vi "Begin.vi"(8 "error in":errorcluster) -> (0 "error out":errorcluster)   [LabVIEW 2014]
doc: "Called before other user functions, this VI is expected to open initial I/O refnums, load in file data, and do all program initialization. Notice that the <B>error out</B> terminal is simply used for data flow. Wiring it to other structures or subVIs ensures that this VI runs first."
uses:
  <vilib>/Rock Robotics/WPI/SafetyOutput/WPI_SafetyOutputConfigMenu.ctl
  <vilib>/Rock Robotics/WPI/DriverStation/WPI_DriverStationRobotMode2.ctl
  <vilib>/Rock Robotics/WPI/Joystick/WPI_JoystickDeviceEnum.ctl
  <vilib>/Rock Robotics/SystemInterfaces/DIO/FPGA_DIOPWMChannel.ctl
  <vilib>/Rock Robotics/SystemInterfaces/AI/FPGA_AIChannel.ctl
  <vilib>/Rock Robotics/SystemInterfaces/Typedef/FPGA_TypedefAnalogModule.ctl
  <vilib>/Rock Robotics/WPI/SerialPort/WPI_SerialPort.ctl
  <vilib>/Rock Robotics/SystemInterfaces/DIO/FPGA_DIOChannel.ctl
  <vilib>/Rock Robotics/WPI/Encoder/WPI_EncoderType.ctl
  Robot Global Data.vi
  <vilib>/Rock Robotics/Network Tables/SD Write String Array.vi
  <vilib>/Rock Robotics/WPI/MotorControl/WPI_MotorControlOpen Talon.vi
  <vilib>/Rock Robotics/WPI/Counter/WPI_CounterDigitalInputToDigitalSource.vi
  <vilib>/Rock Robotics/WPI/RobotDrive/WPI_RobotDriveOpen4MotorWithTalon.vi
  <vilib>/Rock Robotics/SystemInterfaces/spilib/spi_bus.ctl
  <vilib>/Rock Robotics/WPI/SPI/WPI_SPIMode.ctl
  <vilib>/Rock Robotics/SystemInterfaces/Typedef/FPGA_TypedefDigitalModule.ctl
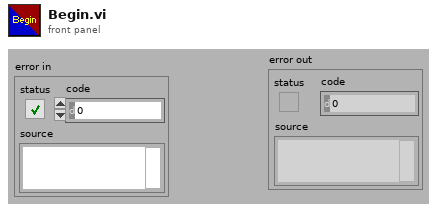
[diagram p1: front panel]
types:
  T1 = typedef "WPI_JoystickDeviceEnum.ctl" = enum16{"USB 0", "USB 1", "USB 2", "USB 3", "USB 4", "USB 5"}
  T2 = typedef "WPI_EncoderType.ctl" = enum16{"1x", "2x", "4x"}
  T3 = typedef "FPGA_DIOChannel.ctl" = enum8{"DIO 0", "DIO 1", "DIO 2", "DIO 3", "DIO 4", "DIO 5", "DIO 6", "DIO 7", "DIO 8", "DIO 9", "DIO MXP 0", "DIO MXP 1", "DIO MXP 2", "DIO MXP 3", "DIO MXP 4", "DIO MXP 5", "DIO MXP 6", "DIO MXP 7", "DIO MXP 8", "DIO MXP 9", "DIO MXP 10", "DIO MXP 11", "DIO MXP 12", "DIO MXP 13", "DIO MXP 14", "DIO MXP 15", "Invalid"}
  T4 = typedef "FPGA_DIOPWMChannel.ctl" = enum8{"PWM 0", "PWM 1", "PWM 2", "PWM 3", "PWM 4", "PWM 5", "PWM 6", "PWM 7", "PWM 8", "PWM 9", "PWM MXP 0", "PWM MXP 1", "PWM MXP 2", "PWM MXP 3", "PWM MXP 4", "PWM MXP 5", "PWM MXP 6", "PWM MXP 7", "PWM MXP 8", "PWM MXP 9", "Invalid"}
  T5 = typedef "WPI_SerialPort.ctl" = enum16{"Onboard RS-232", "MXP TTL"}
  T6 = typedef "FPGA_AIChannel.ctl" = enum8{"AI 0", "AI 1", "AI 2", "AI 3", "AI MXP 0", "AI MXP 1", "AI MXP 2", "AI MXP 3", "Invalid"}
  T7 = typedef "FPGA_TypedefAnalogModule.ctl" = enum16{"Controller 1"}
  T8 = typedef "WPI_DriverStationRobotMode2.ctl" = enum16{"Autonomous Disabled", "Autonomous Enabled", "Teleop Disabled", "Teleop Enabled", "Disconnected", "Finish", "Test Disabled", "Test Enabled", "Emergency Stopped"}
  T9 = typedef "WPI_SafetyOutputConfigMenu.ctl" = enum16{"Enable", "Disable"}
  T10 = typedef "FPGA_TypedefDigitalModule.ctl" = enum16{"Controller 1"}
  T11 = typedef "WPI_SPIMode.ctl" = enum16{"Mode 0 (Clk Idle Low,Sample on Leading)", "Mode 1 (Clk Idle Low,Sample on Trailing)", "Mode 2 (Clk Idle High,Sample on Leading)", "Mode 3 (Clk Idle High,Sample on Trailing)"}
  T12 = typedef "spi_bus.ctl" = enum16{"SPI On-Board, CS0", "SPI On-Board, CS1", "SPI On-Board, CS2", "SPI On-Board, CS3", "SPI MXP", "Invalid"}
  T13 = typedef "WPI_SPIDevRef.ctl" = cluster{"DevStatus":errorcluster, "Handle":i32, "Controller":T10, "SPI Bus":T12}
  T14 = typedef "WPI_SerialPortRef.ctl" = cluster{"DevStatus":errorcluster, "Serial Port Name":refnum<visa-resource-name>}
  T15 = typedef "WPI_DigitalInputDevRef.ctl" = cluster{"DevStatus":errorcluster, "DIO Channel":T3, "Controller":T10}
  T16 = typedef "WPI_JoystickDevRef.ctl" = cluster{"Device":T1}
  T17 = typedef "WPI_RobotDriveDevRef.ctl" = cluster{"DevStatus":errorcluster, "Motors[]":T18[], "Square Inputs":bool, "Max Output":dbl}
  T18 = typedef "WPI_MotorControlDeviceRef.ctl" = cluster{"DeviceStatus":errorcluster, "Type":T19, "PWM":cluster{"Controller":T10, "PWM Channel":T4, "DeadBand":T20}, "CAN":cluster{"Device Number":u8, "Control Mode":T21, "Semaphore":T22, "Max Vout":dbl, "TalonSRX Control Mode":T23}, "Invert":bool, "TransformRef":T24, "InvTransformRef":T24}
  T19 = typedef "WPI_MotorControlType.ctl" = enum16{"PWM", "CAN", "CANTalonSRX"}
  T20 = typedef "WPI_PWMDeadband.ctl" = cluster{"Name":string, "maxPositivePwm":i32, "minPositivePwm":i32, "centerPwm":i32, "maxNegativePwm":i32, "minNegativePwm":i32, "angularRange":u16}
  T21 = typedef "WPI_CANJaguar_ControlMode.ctl" = enum8{"Percent VBus", "Current", "Speed", "Position", "Voltage"}
  T22 = typedef "Semaphore RefNum" = refnum<k1>
  T23 = typedef "WPI_CANTalonSRX_APIControlMode.ctl" = enum8{"Percent VBus", "Speed", "Position", "Slave", "Unchanged / Invalid"}
  T24 = typedef "WPI_PWMTransform_ConPane.ctl" = refnum<vi>
  T25 = typedef "FPGA_CounterEncoderSourceConvertionLVSourceType.ctl" = cluster{"DevStatus":errorcluster, "AnalogTriggerMode?":bool, "DigitalMode":cluster{"Controller":T10, "DIO Channel":T26}, "AnalogTriggerMode":cluster{"AnalogTriggerIndex":T27, "OutputType":T28}}
  T26 = typedef "FPGA_DIODigitalSourceChannel.ctl" = enum8{"DIO 0", "DIO 1", "DIO 2", "DIO 3", "DIO 4", "DIO 5", "DIO 6", "DIO 7", "DIO 8", "DIO 9", "DIO MXP 0", "DIO MXP 1", "DIO MXP 2", "DIO MXP 3", "DIO MXP 4", "DIO MXP 5", "DIO MXP 6", "DIO MXP 7", "DIO MXP 8", "DIO MXP 9", "DIO MXP 10", "DIO MXP 11", "DIO MXP 12", "DIO MXP 13", "DIO MXP 14", "DIO MXP 15", "Disabled"}
  T27 = typedef "FPGA_AnalogTriggerIndex.ctl" = enum8{"Trig 0", "Trig 1", "Trig 2", "Trig 3", "Trig 4", "Trig 5", "Trig 6", "Trig 7", "Invalid"}
  T28 = typedef "FPGA_AnalogTriggerOutType.ctl" = enum16{"InWindow", "TriggerState", "Rising", "Falling"}
  T29 = typedef "WPI_EncoderDevRef.ctl" = cluster{"DevStatus":errorcluster, "EncoderIndex":T30, "CounterIndex":T31, "DistancePerCount":dbl, "Decoding Type":T2}
  T30 = typedef "FPGA_EncoderIdx.ctl" = enum8{"Enc 0", "Enc 1", "Enc 2", "Enc 3", "Enc 4", "Enc 5", "Enc 6", "Enc 7", "Invalid"}
  T31 = typedef "FPGA_CounterCtrSystemIndex.ctl" = enum8{"Ctr 0", "Ctr 1", "Ctr 2", "Ctr 3", "Ctr 4", "Ctr 5", "Ctr 6", "Ctr 7", "Invalid"}
  T32 = typedef "WPI_PotentiometerDevRef.ctl" = cluster{"DevStatus":errorcluster, "Controller":T7, "Analog Channel":T6, "Invert Output":bool}
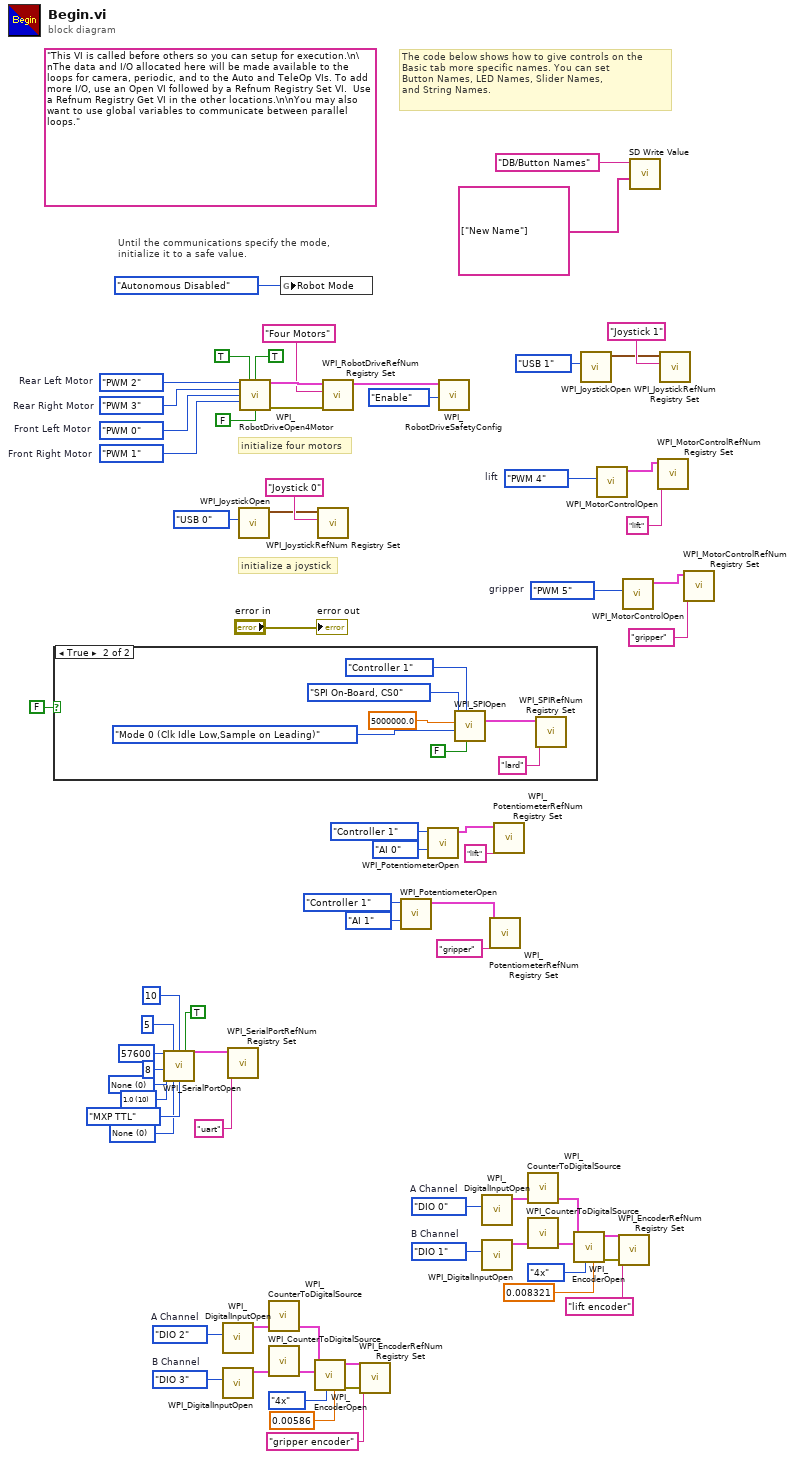
[diagram p0: block diagram]
diagram:
  w19 = FPGA_DIOChannel."DIO 3"  # B Channel
  w18 = FPGA_DIOChannel."DIO 2"  # A Channel
  w29 = FPGA_DIOChannel."DIO 1"  # B Channel
  w28 = FPGA_DIOChannel."DIO 0"  # A Channel
  w32 = FPGA_DIOPWMChannel."PWM 5"  # gripper
  w35 = FPGA_DIOPWMChannel."PWM 4"  # lift
  w38 = u16 0 items=["None", "XON/XOFF", "RTS/CTS", "XON/XOFF & RTS/CTS", "DTR/DSR", "XON/XOFF & DTR/DSR"] ("Flow Control")
  w42 = u16 10 items=["1.0"=10, "1.5"=15, "2.0"=20] ("Stop Bits")
  w43 = u16 0 items=["None", "Odd", "Even", "Mark", "Space"] ("Parity")
  w58 = FPGA_DIOPWMChannel."PWM 1"  # Front Right Motor
  w59 = FPGA_DIOPWMChannel."PWM 0"  # Front Left Motor
  w60 = FPGA_DIOPWMChannel."PWM 3"  # Rear Right Motor
  w61 = FPGA_DIOPWMChannel."PWM 2"  # Rear Left Motor
  (unwired) "This VI is called before others so you can setup for execution.\n\nThe data and I/O allocated here will be made available to the loops for camera, periodic, and to the Auto and TeleOp VIs. To add more I/O, use an Open VI followed by a Refnum Registry Set VI.  Use a Refnum Registry Get VI in the other locations.\n\nYou may also want to use global variables to communicate between parallel loops."
  # "The code below shows how to give controls on the\nBasic tab more specific names. You can set\nButton Names, LED Names, Slider Names,\nand String Names."
  # "initialize a joystick"
  # "Until the communications specify the mode,\ninitialize it to a safe value."
  # "initialize four motors"
  n1 = case shown="True" FALSE {
    frame False {
    }
    frame True {
      n2 = call <vilib>:"WPI_SPIOpen.vi"("Chip Select Active High (F)"=FALSE, "Controller"=FPGA_TypedefDigitalModule."Controller 1", "Mode (3)"=WPI_SPIMode."Mode 0 (Clk Idle Low,Sample on Leading)", "Clock Rate (Hz)"=5000000.0, "SPI Bus"=spi_bus."SPI On-Board, CS0") -> ("SPIDevRef"=w72:T13)  [unwired: 5 in, 1 out]
      n3 = call <vilib>:"WPI_SPIRefNum Registry Set.vi"("refnum name"="lard", "SPIDevRef"=w72) -> ()  [unwired: 8 in, 2 out]
    }
  }
  n4 = call <vilib>:"WPI_SerialPortOpen.vi"("Baud Rate"=u32 57600, "Timeout Value (ms)"=u32 5, "Termination Char (0xA = '\\n' = LF)"=u8 10 ("Termination Char (0xA = '\\n' = LF)"), "Enable Termination Char? (T)"=TRUE, "Data Bits"=u16 8, "Parity"=w43, "Stop Bits"=w42, "Flow Control"=w38, "Serial Port"=WPI_SerialPort."MXP TTL") -> ("SerialPortRef"=w41:T14)  [unwired: 5 in, 1 out]
  n5 = call <vilib>:"WPI_DigitalInputOpen.vi"("DIO Channel"=w18) -> ("DigitalInputDevRef"=w15:T15)  [unwired: 2 in, 8 out]
  n6 = call <vilib>:"WPI_DigitalInputOpen.vi"("DIO Channel"=w19) -> ("DigitalInputDevRef"=w16:T15)  [unwired: 2 in, 8 out]
  n7 = call <vilib>:"WPI_SerialPortRefNum Registry Set.vi"("refnum name"="uart", "SerialPortRef"=w41) -> ()  [unwired: 8 in, 2 out]
  n8 = call <vilib>:"WPI_JoystickOpen.vi"("JoystickDevice"=WPI_JoystickDeviceEnum."USB 0") -> ("JoystickDevRef"=w63:T16)  [unwired: 10 in]
  n9 = call-poly <vilib>:"WPI_RobotDriveOpen4Motor.vi"("Rear Left Motor"=w61, "Rear Left Motor Inverted"=TRUE, "Rear Right Motor Inverted"=TRUE, "Rear Right Motor"=w60, "Front Left Motor"=w59, "Front Right Motor"=w58, "Front Right Motor Inverted"=FALSE) -> ("RobotDriveDevRef"=w70:T17, "error out"=w68:errorcluster)  [unwired: 7 in]
  n10 = call-poly <vilib>:"WPI_CounterToDigitalSource.vi"("DigitalInputDevRef"=w15) -> ("Digital Source"=w14:T25)  [unwired: 6 out]
  n11 = call-poly <vilib>:"WPI_CounterToDigitalSource.vi"("DigitalInputDevRef"=w16) -> ("Digital Source"=w17:T25)  [unwired: 6 out]
  n12 = global write "Robot Global Data.vi" "Robot Mode"(WPI_DriverStationRobotMode2."Autonomous Disabled" ("Robot Mode")) -> ()
  n13 = call <vilib>:"WPI_EncoderOpen.vi"("DistancePerCount"=0.00586, "Decoding Type"=WPI_EncoderType."4x", "BSource"=w17, "ASource"=w14) -> ("error out"=w13:errorcluster, "EncoderDevRef"=w12:T29)  [unwired: 4 in, 2 out]
  n14 = call <vilib>:"WPI_JoystickRefNum Registry Set.vi"("refnum name"="Joystick 0", "JoystickDevRef"=w63) -> ()  [unwired: 8 in, 2 out]
  n15 = call <vilib>:"WPI_RobotDriveRefNum Registry Set.vi"("error in (no error)"=w68, "refnum name"="Four Motors", "RobotDriveDevRef"=w70) -> ("RobotDriveDevRef"=w67:T17)  [unwired: 8 out]
  n16 = call <vilib>:"WPI_EncoderRefNum Registry Set.vi"("error in (no error)"=w13, "refnum name"="gripper encoder", "EncoderDevRef"=w12) -> ()  [unwired: 7 in, 2 out]
  n17 = call <vilib>:"WPI_PotentiometerOpen.vi"("Analog Channel"=FPGA_AIChannel."AI 1", "Controller"=FPGA_TypedefAnalogModule."Controller 1") -> ("PotDevRef"=w50:T32)  [unwired: 8 in, 1 out]
  n18 = call <vilib>:"WPI_PotentiometerOpen.vi"("Analog Channel"=FPGA_AIChannel."AI 0", "Controller"=FPGA_TypedefAnalogModule."Controller 1") -> ("PotDevRef"=w54:T32)  [unwired: 8 in, 1 out]
  n19 = call <vilib>:"WPI_RobotDriveSafetyConfig.vi"("mode"=WPI_SafetyOutputConfigMenu."Enable", "RobotDriveDevRef"=w67) -> ()  [unwired: 8 in, 2 out]
  n20 = call <vilib>:"WPI_DigitalInputOpen.vi"("DIO Channel"=w28) -> ("DigitalInputDevRef"=w25:T15)  [unwired: 2 in, 8 out]
  n21 = call <vilib>:"WPI_DigitalInputOpen.vi"("DIO Channel"=w29) -> ("DigitalInputDevRef"=w26:T15)  [unwired: 2 in, 8 out]
  n22 = call <vilib>:"WPI_PotentiometerRefNum Registry Set.vi"("refnum name"="gripper", "PotDevRef"=w50) -> ()  [unwired: 8 in, 2 out]
  n23 = call <vilib>:"WPI_PotentiometerRefNum Registry Set.vi"("refnum name"="lift", "PotDevRef"=w54) -> ()  [unwired: 8 in, 2 out]
  n24 = call-poly <vilib>:"WPI_CounterToDigitalSource.vi"("DigitalInputDevRef"=w25) -> ("Digital Source"=w24:T25)  [unwired: 6 out]
  n25 = call-poly <vilib>:"WPI_CounterToDigitalSource.vi"("DigitalInputDevRef"=w26) -> ("Digital Source"=w27:T25)  [unwired: 6 out]
  n26 = call <vilib>:"WPI_EncoderOpen.vi"("DistancePerCount"=0.008321, "Decoding Type"=WPI_EncoderType."4x", "BSource"=w27, "ASource"=w24) -> ("error out"=w23:errorcluster, "EncoderDevRef"=w22:T29)  [unwired: 4 in, 2 out]
  n27 = call <vilib>:"WPI_JoystickOpen.vi"("JoystickDevice"=WPI_JoystickDeviceEnum."USB 1") -> ("JoystickDevRef"=w5:T16)  [unwired: 10 in]
  n28 = call-poly <vilib>:"WPI_MotorControlOpen.vi"("PWM Channel"=w35) -> ("MotorControlDeviceRef"=w34:T18)  [unwired: 9 in, 1 out]
  n29 = call <vilib>:"WPI_EncoderRefNum Registry Set.vi"("error in (no error)"=w23, "refnum name"="lift encoder", "EncoderDevRef"=w22) -> ()  [unwired: 7 in, 2 out]
  n30 = call-poly <vilib>:"WPI_MotorControlOpen.vi"("PWM Channel"=w32) -> ("MotorControlDeviceRef"=w31:T18)  [unwired: 9 in, 1 out]
  n31 = call-poly <vilib>:"SD Write Value.vi"("String Array"=string[] ["New Name"], "Name"="DB/Button Names") -> ()  [unwired: 8 in, 2 out]
  n32 = call <vilib>:"WPI_MotorControlRefNum Registry Set.vi"("refnum name"="lift", "MotorControlDevRef"=w34) -> ()  [unwired: 8 in, 2 out]
  n33 = call <vilib>:"WPI_JoystickRefNum Registry Set.vi"("refnum name"="Joystick 1", "JoystickDevRef"=w5) -> ()  [unwired: 8 in, 2 out]
  n34 = call <vilib>:"WPI_MotorControlRefNum Registry Set.vi"("refnum name"="gripper", "MotorControlDevRef"=w31) -> ()  [unwired: 8 in, 2 out]
  "error out" <- "error in"
